vi "Configure.vi"(8 "error in (no error)":errorcluster, 11 "S Parameter in":refnum<class "S Parameter.lvclass">) -> (0 "error out":errorcluster, 3 "S Parameter out":refnum<class "S Parameter.lvclass">)   [LabVIEW 2020, in "S Parameter.lvclass"]
doc: "Configure the measurements paramaters to sweep.\nThis should be a pop up interface invoked by the configure test button on the main panel."
uses:
  S Parameter.lvclass
  S Parameter.lvclass/S Parameter.ctl
panel:
  in  "(De-)Embed":T1(array[cluster])=[{"enabled"=FALSE, "De-embed"=TRUE, "Swap Ports Left"=FALSE, "De-embedding file"=path ""}, {"enabled"=FALSE, "De-embed"=TRUE, "Swap Ports Left"=FALSE, "De-embedding file"=path ""}]
  in  "MDIF-format":bool
  in  "Cancel Button":bool
  in  "VNA ports":bool[](array[boolean])=[TRUE, FALSE, FALSE, FALSE]
  in  "OK Button":bool
  in  "User Note":string
  # "Will use the VNA as is. Need to calibrate the VNA prior to running the measurement"
  # "Left\n\n\n\nRight"
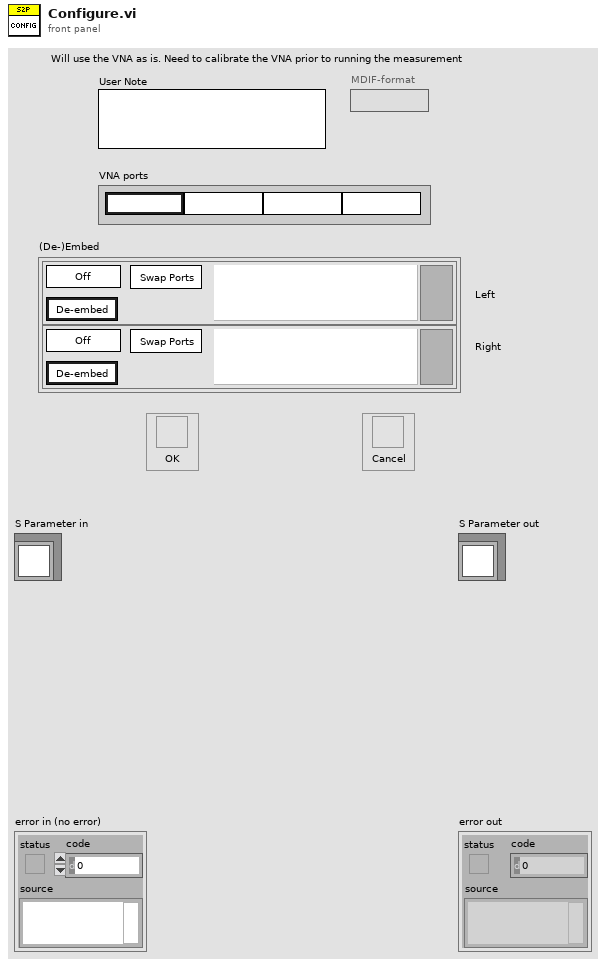
[diagram p1: front panel]
types:
  T1 = cluster{"enabled":bool, "De-embed":bool, "Swap Ports Left":bool, "De-embedding file":path}[]
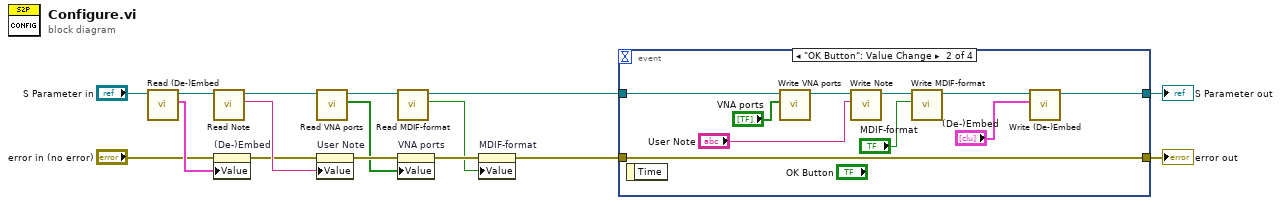
[diagram p0: block diagram]
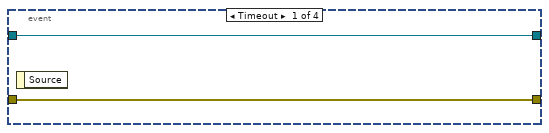
[diagram p2: hidden frame]
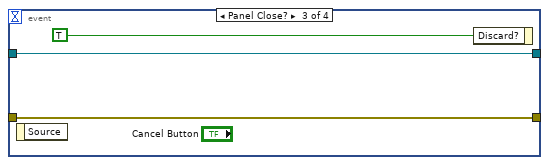
[diagram p3: hidden frame]
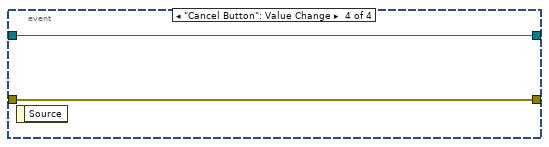
[diagram p4: hidden frame]
diagram:
  n1 = call-dynamic "Read (De-)Embed.vi"("S Parameter in"="S Parameter in") -> ("(De-)Embed"=w3:T1, "S Parameter out"=w4:refnum<class "S Parameter.lvclass">)  [unwired: 9 in]
  n2 = call "Read Note.vi"("S Parameter in"=w4) -> ("Note"=w15:string, "S Parameter out"=w9:refnum<class "S Parameter.lvclass">)  [unwired: 9 in]
  n3 = property on="(De-)Embed" class="Arr"(error in="error in (no error)", "Value"=w3) -> (error out=w1:errorcluster)  [unwired: 1 in, 1 out]
  n4 = call-dynamic "Read VNA ports.vi"("S Parameter in"=w9) -> ("VNA ports"=w7:bool[], "S Parameter out"=w10:refnum<class "S Parameter.lvclass">)  [unwired: 9 in]
  n5 = property on="User Note" class="Str"(error in=w1, "Value"=w15) -> (error out=w11:errorcluster)  [unwired: 1 in, 1 out]
  n6 = call-dynamic "Read MDIF-format.vi"("S Parameter in"=w10) -> ("MDIF-format"=w6:bool, "S Parameter out"=w8:refnum<class "S Parameter.lvclass">)  [unwired: 9 in]
  n7 = property on="VNA ports" class="Arr (strict)"(error in=w11, "Value"=w7) -> (error out=w13:errorcluster)  [unwired: 1 in, 1 out]
  n8 = property on="MDIF-format" class="Bool (strict)"(error in=w13, "Value"=w6) -> (error out=w12:errorcluster)  [unwired: 1 in, 1 out]
  n9 = event shown="[1] \"OK Button\": Value Change" {
    selector: _ -> [_ _ _ _]
    dyn-events: _ -> [_ _ _ _]
    timeout: _ -> [_ _ _ _]
    tunnel: w12 -> [w18 w28 w30 w33]
    tunnel: [w18 w28 w30 w33] -> w16
    tunnel: w8 -> [w17 w25 w29 w32]
    tunnel: [w17 w20 w29 w32] -> w14
    event Timeout {
      n10 = event-data() -> ()  [unwired: 1 in, 1 out]
    }
    event "OK Button": Value Change {
      n11 = event-data() -> ()  [unwired: 1 in, 1 out]
      n12 = call-dynamic "Write VNA ports.vi"("VNA ports"="VNA ports", "S Parameter in"=w25) -> ("S Parameter out"=w27:refnum<class "S Parameter.lvclass">)  [unwired: 9 in]
      n13 = call "Write Note.vi"("Note"="User Note", "S Parameter in"=w27) -> ("S Parameter out"=w23:refnum<class "S Parameter.lvclass">)  [unwired: 9 in]
      n14 = call-dynamic "Write MDIF-format.vi"("MDIF-format"="MDIF-format", "S Parameter in"=w23) -> ("S Parameter out"=w21:refnum<class "S Parameter.lvclass">)  [unwired: 9 in]
      n15 = call-dynamic "Write (De-)Embed.vi"("(De-)Embed"="(De-)Embed", "S Parameter in"=w21) -> ("S Parameter out"=w20:refnum<class "S Parameter.lvclass">)  [unwired: 9 in]
    }
    event Panel Close? {
      n16 = event-data() -> ()  [unwired: 1 in, 1 out]
      n17 = event-data("Discard?"=TRUE) -> ()  [unwired: 1 in, 1 out]
    }
    event "Cancel Button": Value Change {
      n18 = event-data() -> ()  [unwired: 1 in, 1 out]
    }
  }
  "error out" <- w16
  "S Parameter out" <- w14
